vi "Main On Compile VI_Parse properties.vi"(8 "error in (no error)":errorcluster, 11 "Device Reference":T2 format="%.0x") -> (0 "error out":errorcluster, 1 "Write Block Descriptors":T1[](array[typedef]), 2 "Read Block Descriptors":T1[](array[typedef]), 3 "Device Ref out":T2 format="%.0x", 4 "Write":bool, 5 "max channel count bytes":u32, 6 "Read":bool)   [LabVIEW 2019, in "GE_RM_System Explorer.lvlib"]
uses:
  GE_RM_System Explorer.lvlib
  <vilib>/NI VeriStand/Custom Device API/Custom Device Item Ref.ctl
  Shared/Block descriptor.ctl
  Shared/Data Channel Type.ctl
  Shared/Global.vi
  <vilib>/NI VeriStand/Custom Device API/Get Item Property (U16).vi
  <vilib>/NI VeriStand/Custom Device API/Get Item Property (U32).vi
  Shared/GE_RM_Shared.lvlib
  <vilib>/NI VeriStand/Custom Device API/Custom Device API.lvlib
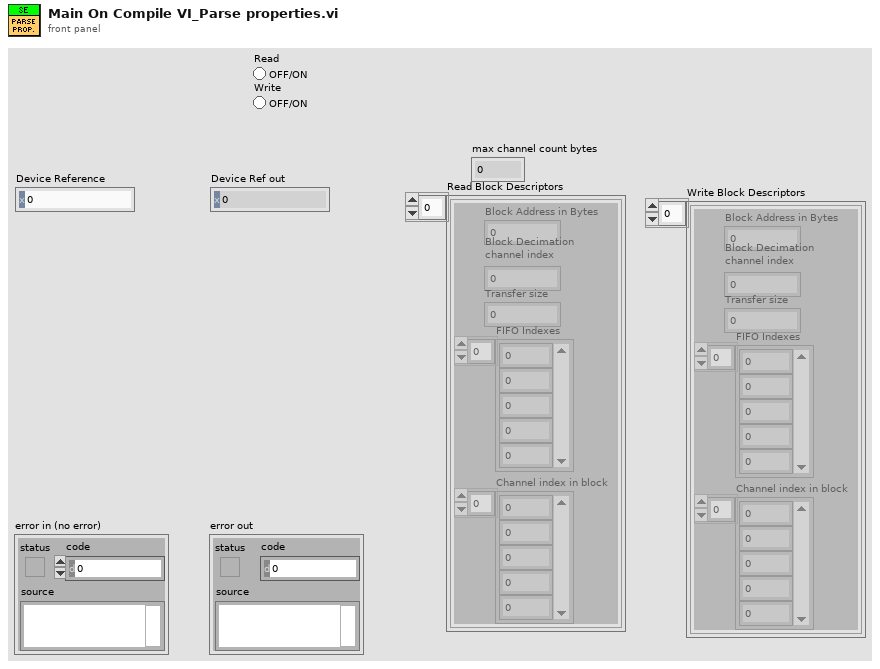
[diagram p1: front panel]
types:
  T1 = typedef "GE_RM_Shared.lvlib/Block descriptor.ctl" = cluster{"Block Address in Bytes":u32, "Block Decimation \nchannel index":i32, "Transfer size":u32, "FIFO Indexes":i32[], "Channel index in block":i32[]}
  T2 = typedef "Custom Device API.lvlib/Custom Device Item Ref.ctl" = u64
  T3 = typedef "GE_RM_System Explorer.lvlib/Data Channel Type.ctl" = enum16{"Read", "Write"}
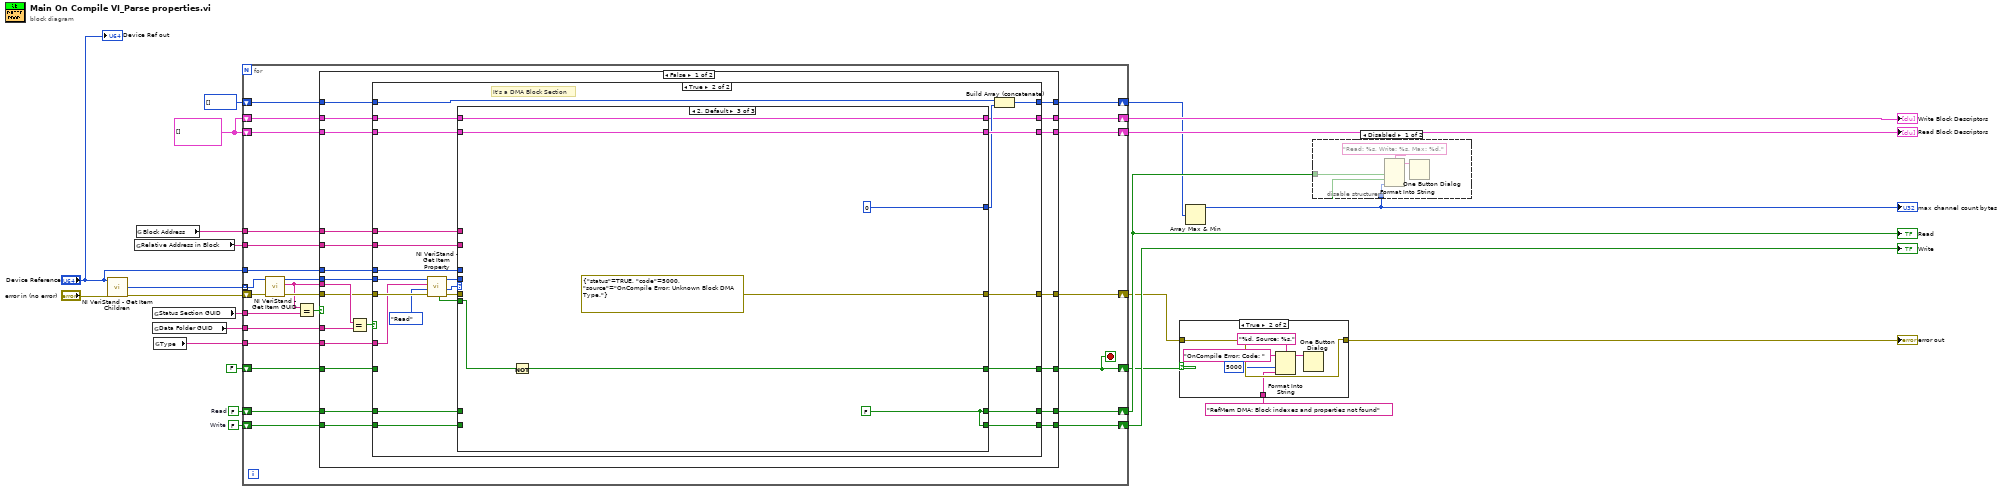
[diagram p0: block diagram]
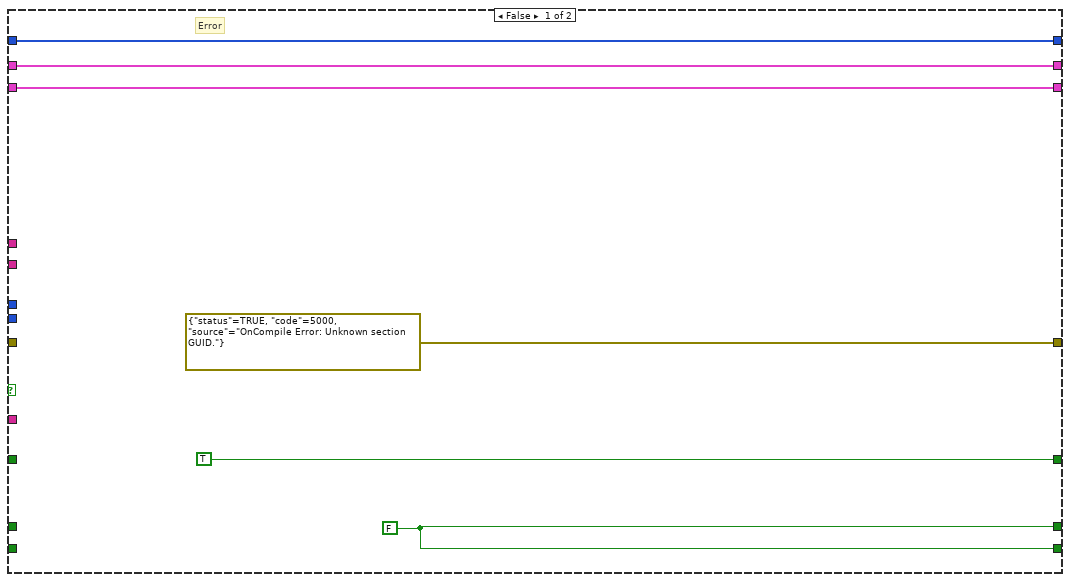
[diagram p2: hidden frame]
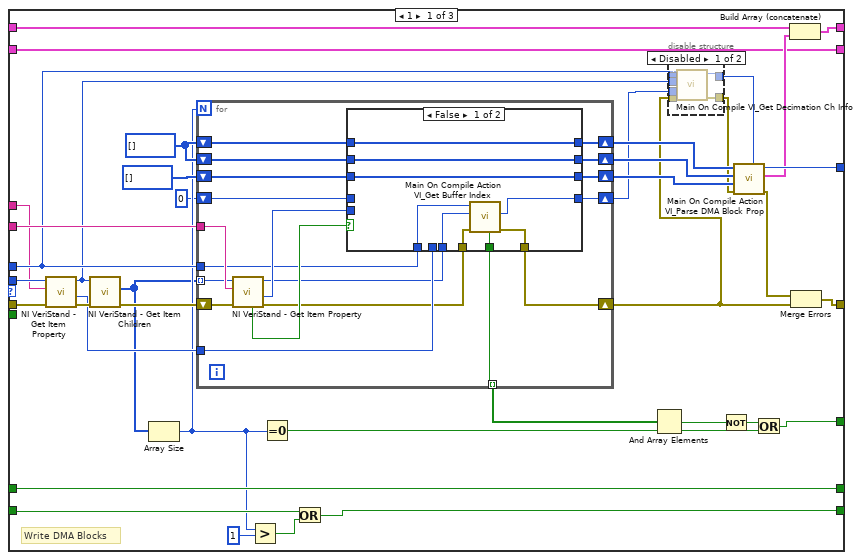
[diagram p3: hidden frame]
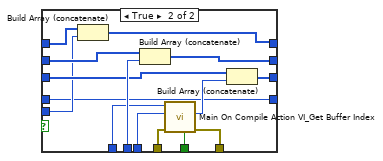
[diagram p5: hidden frame]
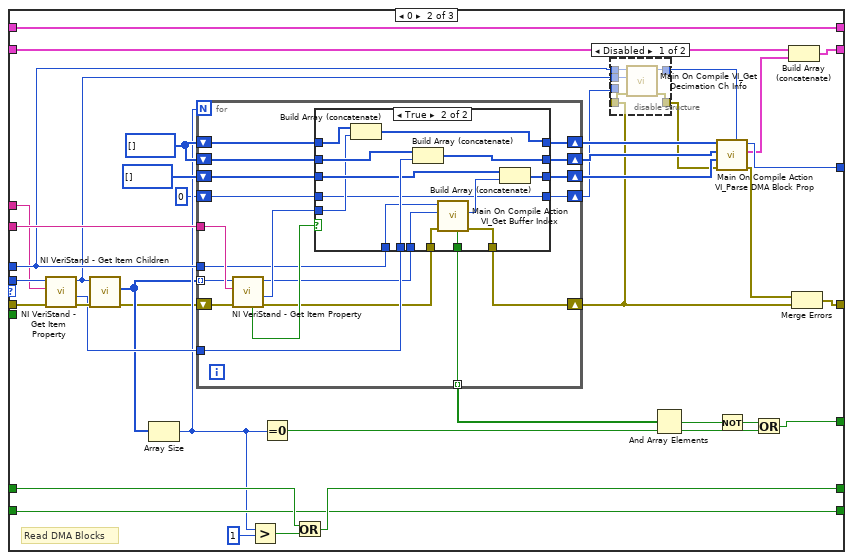
[diagram p6: hidden frame]
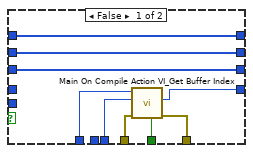
[diagram p8: hidden frame]
diagram:
  w6 = FALSE  # Write
  w7 = FALSE  # Read
  w12 = T1[] [] ("GE_RM_Shared.lvlib:Block descriptor.ctlDMA Blocks")
  n1 = call <vilib>:"NI VeriStand - Get Item Children.vi"("error in (no error)"="error in (no error)", "Item Ref in"="Device Reference") -> ("error out"=w13:errorcluster, "Child Refs"=w1:T2[])  [unwired: 6 in, 2 out]
  n2 = global read "Global.vi" "Relative Address in Block"() -> (w15:string)
  n3 = global read "Global.vi" "Block Address"() -> (w14:string)
  n4 = global read "Global.vi" "Status Section GUID"() -> (w11:string)
  n5 = global read "Global.vi" "Data Folder GUID"() -> (w10:string)
  n6 = global read "Global.vi" "Type"() -> (w4:string)
  n7 = for {
    tunnel: "Device Reference" -> [w47]
    tunnel: w15 -> [w46]
    tunnel: w14 -> [w45]
    tunnel: w1 -> [w43] mode=indexing
    shift-right: [w48] -> w2
    shift-left: w13 -> [w44]
    shift-right: [w49] -> w23
    shift-left: w12 -> [w37]
    shift-right: [w35] -> w20
    shift-left: w12 -> [w36]
    tunnel: w11 -> [w39]
    tunnel: w10 -> [w38]
    shift-right: [w34] -> w3
    shift-left: FALSE -> [w33]
    shift-right: [w32] -> w8
    shift-left: u32[] [] -> [w27]
    shift-right: [w29] -> w22
    shift-left: w7 -> [w31]
    shift-right: [w28] -> w21
    shift-left: w6 -> [w30]
    tunnel: w4 -> [w26]
    stop <- w34 stop-if-true
    n8 = call <vilib>:"NI VeriStand - Get Item GUID.vi"("error in (no error)"=w44, "Item Ref in"=w43) -> ("error out"=w42:errorcluster, "GUID"=w40:string, "Item Ref out"=w25:T2)  [unwired: 7 in]
    n9 = Equal?(x=w40, y=w39) -> (x = y?=w41:bool)
    n10 = case shown="False" w41 {
      tunnel: [w71 w286] -> w49
      tunnel: [w70 w285] -> w48
      tunnel: [w69 w289] -> w34
      tunnel: w47 -> [w68 _]
      tunnel: w46 -> [w67 _]
      tunnel: w45 -> [w66 _]
      tunnel: w42 -> [w52 w285]
      tunnel: w40 -> [w65 _]
      tunnel: w38 -> [w64 _]
      tunnel: w37 -> [w62 w286]
      tunnel: w36 -> [w61 w287]
      tunnel: [w60 w287] -> w35
      tunnel: w33 -> [w59 w289]
      tunnel: [w58 w288] -> w32
      tunnel: w31 -> [w57 w291]
      tunnel: w30 -> [w56 w290]
      tunnel: [w51 w291] -> w29
      tunnel: [w50 w290] -> w28
      tunnel: w27 -> [w55 w288]
      tunnel: w26 -> [w54 _]
      tunnel: w25 -> [w53 _]
      frame False {
        n11 = Equal?(x=w65, y=w64) -> (x = y?=w63:bool)
        n12 = case shown="True" w63 {
          tunnel: [w76 w101] -> w71
          tunnel: [errorcluster {"status"=TRUE, "code"=5000, "source"="OnCompile Error: Unknown section GUID."} ("error IO") w100] -> w70
          tunnel: [TRUE w99] -> w69
          tunnel: w68 -> [_ w98]
          tunnel: w67 -> [_ w97]
          tunnel: w66 -> [_ w96]
          tunnel: w62 -> [w76 w86]
          tunnel: w61 -> [w77 w87]
          tunnel: [w77 w85] -> w60
          tunnel: w59 -> [_ _]
          tunnel: [w75 w94] -> w58
          tunnel: w57 -> [_ w84]
          tunnel: w56 -> [_ w82]
          tunnel: w55 -> [w75 w93]
          tunnel: w54 -> [_ w90]
          tunnel: w53 -> [_ w92]
          tunnel: w52 -> [_ w91]
          tunnel: [w72 w83] -> w51
          tunnel: [w72 w79] -> w50
          frame False {
            w72 = FALSE ("Read")
            # "Error"
          }
          frame True {
            # "It's a DMA Block Section"
            n13 = call-poly <vilib>:"NI VeriStand - Get Item Property.vi"("error in (no error)"=w91, "Default Value"=Data_Channel_Type."Read" ("DataChan Type"), "Property Name"=w90, "Item Ref in"=w92) -> ("error out"=w80:errorcluster, "Value"=w88:u16, "Item Ref out"=w81:T2, "Found?"=w78:bool)  [unwired: 4 in]
            n14 = case shown="2, Default" w88 {
              tunnel: [w125 w204 w283] -> w101
              tunnel: [w139 w227 errorcluster {"status"=TRUE, "code"=5000, "source"="OnCompile Error: Unknown Block DMA Type."} ("error IO")] -> w100
              tunnel: [w138 w226 w278] -> w99
              tunnel: w98 -> [w117 w213 _]
              tunnel: w97 -> [w137 w225 _]
              tunnel: w96 -> [w115 w211 _]
              tunnel: [w128 w216 u32 0 ("max block size")] -> w95
              tunnel: w87 -> [w127 w203 w284]
              tunnel: w86 -> [w125 w206 w283]
              tunnel: [w124 w203 w284] -> w85
              tunnel: w84 -> [w123 w202 _]
              tunnel: [w123 w201 w281] -> w83
              tunnel: w82 -> [w120 w200 _]
              tunnel: w81 -> [w116 w212 _]
              tunnel: w80 -> [w114 w210 _]
              tunnel: [w118 w200 w281] -> w79
              tunnel: w78 -> [_ _ w279]
              frame 1 {
                w132 = u32[] []
                # "Write DMA Blocks"
                n15 = call-poly <vilib>:"NI VeriStand - Get Item Property.vi"("error in (no error)"=w114, "Property Name"=w115, "Item Ref in"=w116) -> ("error out"=w113:errorcluster, "Value"=w112:u32, "Item Ref out"=w106:T2)  [unwired: 5 in, 1 out]
                n16 = call <vilib>:"NI VeriStand - Get Item Children.vi"("error in (no error)"=w113, "Item Ref in"=w106) -> ("error out"=w122:errorcluster, "Child Refs"=w107:T2[])  [unwired: 6 in, 2 out]
                n17 = Array Size(array=w107) -> (size(s)=w108:i32)
                n18 = for {
                  N: w108 -> [_]
                  tunnel: w137 -> [w164]
                  shift-right: [w155] -> w111
                  shift-left: w122 -> [w165]
                  tunnel: w117 -> [w153]
                  tunnel: [w154] -> w110 mode=indexing
                  shift-right: [w160] -> w135
                  shift-left: w132 -> [w163]
                  shift-right: [w159] -> w134
                  shift-left: w132 -> [w162]
                  shift-right: [w158] -> w133
                  shift-left: i32[] [] -> [w161]
                  tunnel: w112 -> [w152]
                  tunnel: w107 -> [w149] mode=indexing
                  shift-right: [w148] -> w104
                  shift-left: 0 ("Channel FIFO Buffer Index") -> [w147]
                  n19 = call-poly <vilib>:"NI VeriStand - Get Item Property.vi"("error in (no error)"=w165, "Property Name"=w164, "Item Ref in"=w149) -> ("error out"=w150:errorcluster, "Value"=w157:u32, "Item Ref out"=w151:T2, "Found?"=w156:bool)  [unwired: 5 in]
                  n20 = case shown="False" w156 {
                    tunnel: [w174 w183] -> w160
                    tunnel: w163 -> [w174 w189]
                    tunnel: [w173 w186] -> w159
                    tunnel: w162 -> [w173 w187]
                    tunnel: [w172 w184] -> w158
                    tunnel: w161 -> [w172 w185]
                    tunnel: w152 -> [_ w188]
                    tunnel: w157 -> [_ w182]
                    tunnel: w150 -> [w169 w181]
                    tunnel: [w170 w180] -> w155
                    tunnel: [w171 w179] -> w154
                    tunnel: w153 -> [w167 w178]
                    tunnel: w151 -> [w166 w177]
                    tunnel: [w168 w175] -> w148
                    tunnel: w147 -> [_ w175]
                    frame False {
                      n21 = call "Main On Compile Action VI_Get Buffer Index.vi"("error in"=w169, "Channel Ref"=w166, "Device Ref in"=w167) -> ("error out"=w170:errorcluster, "Channel FIFO Buffer Index"=w168:i32, "Found"=w171:bool)  [unwired: 4 in, 2 out]
                    }
                    frame True {
                      n22 = Build Array (concatenate)(w189, w182) -> (w183:u32[])
                      n23 = Build Array (concatenate)(w187, w188) -> (w186:u32[])
                      n24 = call "Main On Compile Action VI_Get Buffer Index.vi"("error in"=w181, "Channel Ref"=w177, "Device Ref in"=w178) -> ("error out"=w180:errorcluster, "Channel FIFO Buffer Index"=w176:i32, "Found"=w179:bool)  [unwired: 4 in, 2 out]
                      n25 = Build Array (concatenate)(w185, w176) -> (w184:i32[])
                    }
                  }
                }
                n26 = Greater?(x=w108, y=1) -> (0:w119:bool)
                n27 = Equal To 0?(x=w108) -> (x = 0?=w129:bool)
                n28 = Or(x=w120, y=w119) -> (x .or. y?=w118:bool)
                n29 = And Array Elements(Boolean array=w110) -> (logical AND=w130:bool)
                n30 = disable-structure shown="Disabled" {
                  disable-tunnel: w117 -> [w144 _]
                  disable-tunnel: [w143 w145] -> w103
                  disable-tunnel: [w142 w146] -> w102
                  disable-tunnel: w111 -> [w141 w145]
                  disable-tunnel: w106 -> [w140 _]
                  disable-tunnel: w104 -> [_ w146]
                  frame Disabled {
                    n31 = call "Main On Compile VI_Get Decimation Ch Info.vi"("error in (no error)"=w141, "Section Reference"=w140, "Device Reference"=w144) -> ("error out"=w143:errorcluster, "Decimation FIFO Index"=w142:i32)  [unwired: 7 in]
                  }
                  frame Enabled {
                  }
                }
                n32 = Not(x=w130) -> (.not. x?=w109:bool)
                n33 = call "Main On Compile Action VI_Parse DMA Block Prop.vi"("Decimation FIFO Index"=w102, "error in (no error)"=w103, "FIFO indexes"=w133, "Block Address"=w134, "Relative Address in Block"=w135) -> ("error out"=w136:errorcluster, "Block descriptor"=w126:T1, "max block size"=w128:u32)  [unwired: 4 in]
                n34 = Or(x=w109, y=w129) -> (x .or. y?=w138:bool)
                n35 = Build Array (concatenate)(w127, w126) -> (w124:T1[])
                n36 = Merge Errors(w136, w111) -> (w139:errorcluster)
              }
              frame 0 {
                w221 = u32[] []
                # "Read DMA Blocks"
                n37 = call-poly <vilib>:"NI VeriStand - Get Item Property.vi"("error in (no error)"=w210, "Property Name"=w211, "Item Ref in"=w212) -> ("error out"=w209:errorcluster, "Value"=w208:u32, "Item Ref out"=w196:T2)  [unwired: 5 in, 1 out]
                n38 = call <vilib>:"NI VeriStand - Get Item Children.vi"("error in (no error)"=w209, "Item Ref in"=w196) -> ("error out"=w193:errorcluster, "Child Refs"=w197:T2[])  [unwired: 6 in, 2 out]
                n39 = Array Size(array=w197) -> (size(s)=w198:i32)
                n40 = for {
                  N: w198 -> [_]
                  tunnel: w225 -> [w252]
                  shift-right: [w243] -> w192
                  shift-left: w193 -> [w253]
                  tunnel: w213 -> [w241]
                  tunnel: [w242] -> w207 mode=indexing
                  shift-right: [w248] -> w224
                  shift-left: w221 -> [w251]
                  shift-right: [w247] -> w223
                  shift-left: w221 -> [w250]
                  shift-right: [w246] -> w222
                  shift-left: i32[] [] -> [w249]
                  tunnel: w208 -> [w240]
                  tunnel: w197 -> [w237] mode=indexing
                  shift-right: [w236] -> w194
                  shift-left: 0 ("Channel FIFO Buffer Index") -> [w235]
                  n41 = call-poly <vilib>:"NI VeriStand - Get Item Property.vi"("error in (no error)"=w253, "Property Name"=w252, "Item Ref in"=w237) -> ("error out"=w238:errorcluster, "Value"=w245:u32, "Item Ref out"=w239:T2, "Found?"=w244:bool)  [unwired: 5 in]
                  n42 = case shown="True" w244 {
                    tunnel: [w262 w271] -> w248
                    tunnel: w251 -> [w262 w277]
                    tunnel: [w261 w274] -> w247
                    tunnel: w250 -> [w261 w275]
                    tunnel: [w260 w272] -> w246
                    tunnel: w249 -> [w260 w273]
                    tunnel: w240 -> [_ w276]
                    tunnel: w245 -> [_ w270]
                    tunnel: w238 -> [w257 w269]
                    tunnel: [w258 w268] -> w243
                    tunnel: [w259 w267] -> w242
                    tunnel: w241 -> [w256 w266]
                    tunnel: w239 -> [w255 w265]
                    tunnel: [w254 w263] -> w236
                    tunnel: w235 -> [_ w263]
                    frame False {
                      n43 = call "Main On Compile Action VI_Get Buffer Index.vi"("error in"=w257, "Channel Ref"=w255, "Device Ref in"=w256) -> ("error out"=w258:errorcluster, "Channel FIFO Buffer Index"=w254:i32, "Found"=w259:bool)  [unwired: 4 in, 2 out]
                    }
                    frame True {
                      n44 = Build Array (concatenate)(w277, w270) -> (w271:u32[])
                      n45 = Build Array (concatenate)(w275, w276) -> (w274:u32[])
                      n46 = call "Main On Compile Action VI_Get Buffer Index.vi"("error in"=w269, "Channel Ref"=w265, "Device Ref in"=w266) -> ("error out"=w268:errorcluster, "Channel FIFO Buffer Index"=w264:i32, "Found"=w267:bool)  [unwired: 4 in, 2 out]
                      n47 = Build Array (concatenate)(w273, w264) -> (w272:i32[])
                    }
                  }
                }
                n48 = Greater?(x=w198, y=1) -> (0:w214:bool)
                n49 = Equal To 0?(x=w198) -> (x = 0?=w217:bool)
                n50 = Or(x=w202, y=w214) -> (x .or. y?=w201:bool)
                n51 = disable-structure shown="Disabled" {
                  disable-tunnel: w213 -> [w232 _]
                  disable-tunnel: w196 -> [w231 _]
                  disable-tunnel: w192 -> [w230 w234]
                  disable-tunnel: [w229 w233] -> w191
                  disable-tunnel: [w228 w234] -> w190
                  disable-tunnel: w194 -> [_ w233]
                  frame Disabled {
                    n52 = call "Main On Compile VI_Get Decimation Ch Info.vi"("error in (no error)"=w230, "Section Reference"=w231, "Device Reference"=w232) -> ("error out"=w228:errorcluster, "Decimation FIFO Index"=w229:i32)  [unwired: 7 in]
                  }
                  frame Enabled {
                  }
                }
                n53 = And Array Elements(Boolean array=w207) -> (logical AND=w218:bool)
                n54 = call "Main On Compile Action VI_Parse DMA Block Prop.vi"("Decimation FIFO Index"=w191, "error in (no error)"=w190, "FIFO indexes"=w222, "Block Address"=w223, "Relative Address in Block"=w224) -> ("error out"=w219:errorcluster, "Block descriptor"=w205:T1, "max block size"=w216:u32)  [unwired: 4 in]
                n55 = Not(x=w218) -> (.not. x?=w199:bool)
                n56 = Or(x=w199, y=w217) -> (x .or. y?=w226:bool)
                n57 = Build Array (concatenate)(w206, w205) -> (w204:T1[])
                n58 = Merge Errors(w219, w192) -> (w227:errorcluster)
              }
              frame 2, Default {
                w281 = FALSE ("Read")
                n59 = Not(x=w279) -> (.not. x?=w278:bool)
              }
            }
            n60 = Build Array (concatenate)(w93, w95) -> (w94:u32[])
          }
        }
      }
      frame True {
      }
    }
  }
  "Read Block Descriptors" <- w23
  "Read" <- w22
  "Write" <- w21
  "Write Block Descriptors" <- w20
  n61 = case shown="True" w3 {
    tunnel: [w292 w298] -> w24
    tunnel: w2 -> [w292 w298]
    tunnel: "RefMem DMA: Block indexes and properties not found" ("error message (\"\")") -> [_ w295]
    frame False {
    }
    frame True {
      n62 = Format Into String(format string="%d, Source: %s.", initial string="OnCompile Error: Code: ", 5000 ("error code (0)"), w295) -> (resulting string=w297:string)  [unwired: 1 in, 1 out]
      n63 = One Button Dialog(message=w297) -> ()  [unwired: 1 in, 1 out]
    }
  }
  "error out" <- w24
  n64 = Array Max & Min(array=w8) -> (max value=w19:u32)  [unwired: 3 out]
  "max channel count bytes" <- w19
  n65 = disable-structure shown="Disabled" {
    disable-tunnel: w22 -> [w300 _]
    disable-tunnel: w19 -> [w299 _]
    frame Disabled {
      n66 = Format Into String(format string="Read: %s, Write: %s, Max: %d.", w300, w300, w299) -> (resulting string=w302:string)  [unwired: 2 in, 1 out]
      n67 = One Button Dialog(message=w302) -> ()  [unwired: 1 in, 1 out]
    }
    frame Enabled {
    }
  }
  "Device Ref out" <- "Device Reference"
